vi "Evaluate Destination Subpanel.vi"(9 "Destination Subpanel":T1, 11 "Viewable in":refnum<class "IViewable.lvclass">) -> (2 "Already Inserted?":bool)   [LabVIEW 2020, in "IViewable.lvlib" / "IViewable.lvclass"]
doc: "评估目标子面板"
uses:
  IViewable.lvclass
  ProtectedSubpanel/Protected Subpanel Reference.ctl
  ProtectedSubpanel/ProtectedSubpanel.lvclass
  IViewable.lvclass/IViewable.ctl
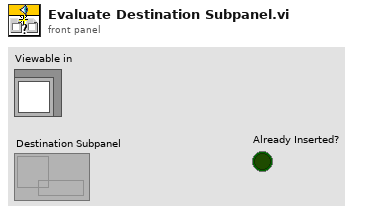
[diagram p1: front panel]
types:
  T1 = typedef "IViewable.lvlib/ProtectedSubpanel.lvclass/Protected Subpanel Reference.ctl" = refnum<data-value>
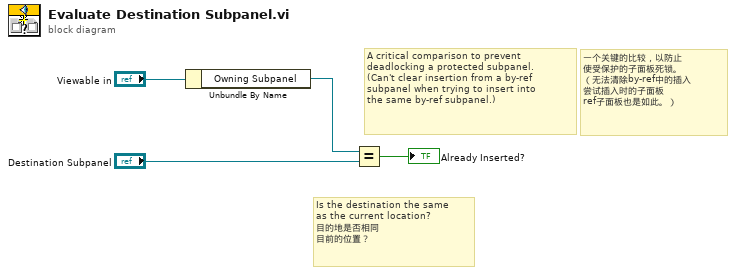
[diagram p0: block diagram]
diagram:
  # "一个关键的比较，以防止\n使受保护的子面板死锁。 \n（无法清除by-ref中的插入\n尝试插入时的子面板\nref子面板也是如此。）"
  # "Is the destination the same\nas the current location?\n目的地是否相同\n目前的位置？"
  # "A critical comparison to prevent\ndeadlocking a protected subpanel. \n(Can't clear insertion from a by-ref\nsubpanel when trying to insert into\nthe same by-ref subpanel.)"
  n1 = Unbundle By Name("Viewable in") -> ("Owning Subpanel"=w3:T1)
  n2 = Equal?(x=w3, y="Destination Subpanel") -> (x = y?=→"Already Inserted?":bool)
